vi "Probes - Equations.vi"() -> ()   [LabVIEW 2015]
panel:
  out "x2":dbl=-5.0
  out "x1":dbl=3.0
  in  "c":dbl=-15.0
  in  "b":dbl=2.0
  in  "a":dbl=1.0
  # "When\na = 1\nb = -5\nc = -24\n\nx1 = 8\nx2 = -3"
  # "When\na = 3\nb = 5\nc = -7\n\nx1 = 0.907\nx2 = -2.573"
  # "When\na = -1\nb = -6\nc = 8\n\nx1 = -7.123\nx2 = 1.123"
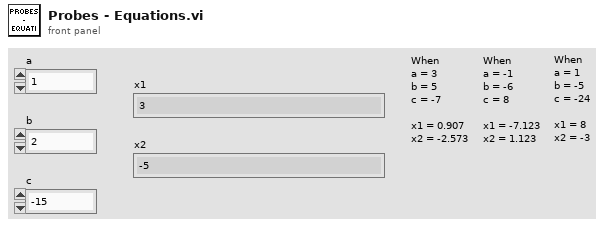
[diagram p1: front panel]
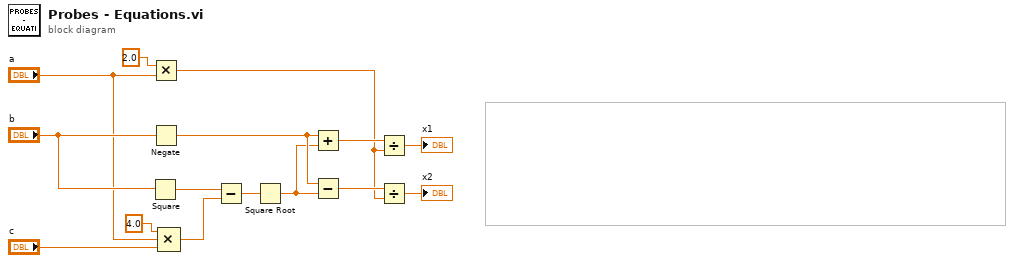
[diagram p0: block diagram]
diagram:
  n1 = Square(x="b") -> (x^2=w4:dbl)
  n2 = Multiply(x=2.0 ("n"), y="a") -> (x*y=w2:dbl)
  n3 = Negate(x="b") -> (-x=w11:dbl)
  n4 = Compound Arithmetic op=MULTIPLY(4.0, "a", "c") -> (w14:dbl)
  n5 = Subtract(x=w4, y=w14) -> (x-y=w6:dbl)
  n6 = Square Root(x=w6) -> (sqrt(x)=w7:dbl)
  n7 = Add(x=w11, y=w7) -> (x+y=w13:dbl)
  n8 = Subtract(x=w11, y=w7) -> (x-y=w10:dbl)
  n9 = Divide(x=w13, y=w2) -> (x/y=→"x1":dbl)
  n10 = Divide(x=w10, y=w2) -> (x/y=→"x2":dbl)
